vi "Demo - Hardware in the Loop Application.vi"() -> ()   [LabVIEW 2017]
doc: "This application demonstrates the basic application of the hardware in the loop mode.\n\n-Initialises and configures the device\n-Uploads data the arbitrary waveform generator\n-Runs a shot\n-Downloads the data and displays it\n-Changes the data\n-Repeats the process"
uses:
  Communications/Typedefs/Data Size--Enum.ctl
  Communications/Communications Library.lvlib
  GUI/Consoles/Communications Console Library.lvlib
panel:
  in  "Analog In Data Size":T1
  in  "Display Console":bool
  in  "INI File Path":path caption="INI File Path (Blank for Defaults)"
  out "Ready":bool
  out "error out":errorcluster
  out "Number of Shots Run":i32
  in  "stop":bool
  in  "Dynamic Channel":i32
  in  "Speed":dbl=0.5 format="%#_13g"
  out "Data Received":bool
  out "Shot Completed":bool
  in  "Samples to Read":i32=80000
  in  "Length of AO Data (Samples)":i32=32768
  out "Analog Input Plot":i32[][](graph)
  out "Analog Output Plot":i16[][](graph)
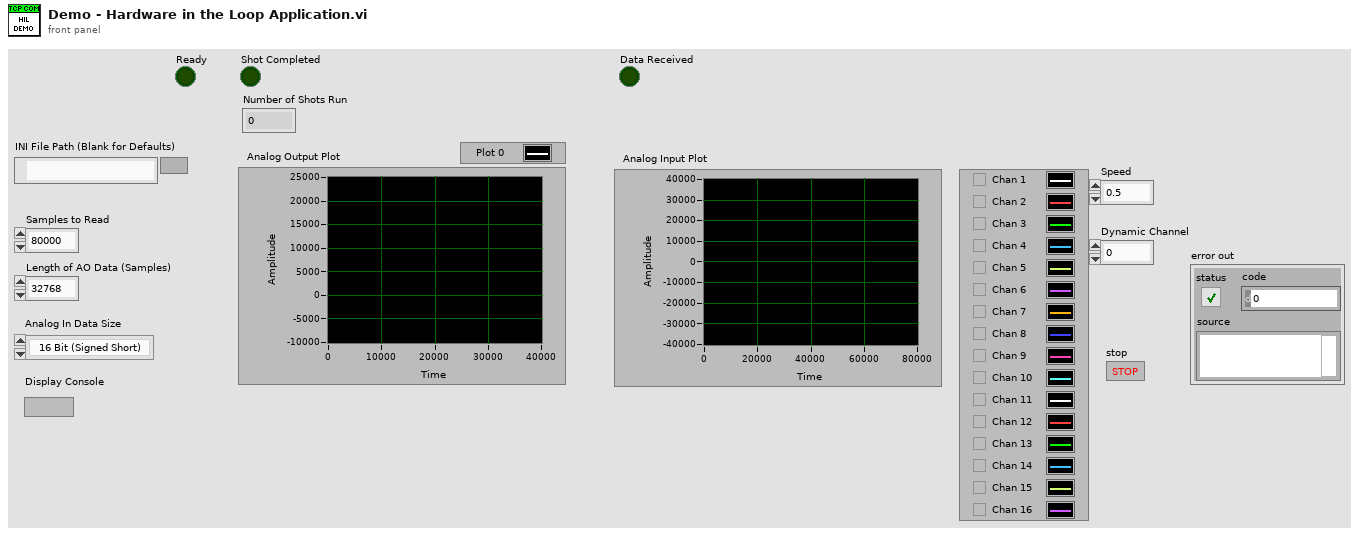
[diagram p1: front panel]
types:
  T1 = typedef "Communications Library.lvlib/Data Size--Enum.ctl" = enum16{"16 Bit (Signed Short)", "32 Bit (Signed Long)"}
  T2 = typedef "Communications Library.lvlib/DTACQ Module Carrier Configuration--Cluster.ctl" = cluster{"Name":string, "IP":string, "Control Port":i32, "Timeout (ms)":i32, "Continuous Capture Port (Multiplexed)":i32, "Start HIL Shot Port":i32, "AWG Upload Port (Multiplexed)":i32, "Download Captured Data Port (Multiplexed)":i32, "Module Slots":i32, "Module Configurations":T3[]}
  T3 = typedef "Communications Library.lvlib/DTACQ Module Configuration--Cluster.ctl" = cluster{"Name":string, "Position":string, "Module Type":T4, "Control Port":i32, "Timeout (ms)":i32, "Channels":i32}
  T4 = typedef "Communications Library.lvlib/DTACQ Device Type--Enum.ctl" = enum16{"Carrier", "Analog In Module", "Analog Out Module", "Generic Module"}
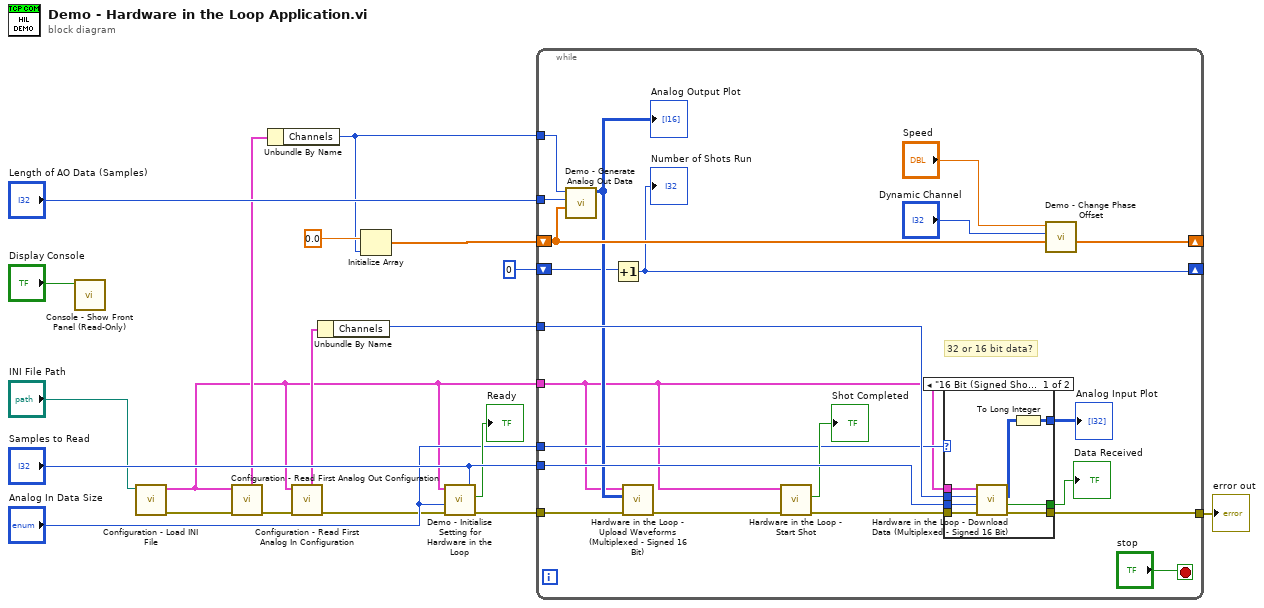
[diagram p0: block diagram]
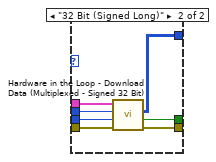
[diagram p2: hidden frame]
diagram:
  n1 = call "Console - Show Front Panel (Read-Only).vi"("Display Console"="Display Console") -> ()  [unwired: 11 in]
  n2 = call "Configuration - Load INI File.vi"("configuration file path"="INI File Path") -> ("error out"=w12:errorcluster, "Carrier Configuration Out"=w1:T2)  [unwired: 9 in]
  n3 = call "Configuration - Read First Analog Out Configuration.vi"("error in"=w12, "Configuration Cluster"=w1) -> ("error out"=w11:errorcluster, "AO - Module Configuration"=w10:T3)  [unwired: 5 in, 3 out]
  n4 = Unbundle By Name(w10) -> ("Channels"=w9:i32)
  n5 = call "Configuration - Read First Analog In Configuration.vi"("error in"=w11, "Carrier Configuration"=w1) -> ("error out"=w2:errorcluster, "AI - Module Configuration"=w8:T3)  [unwired: 5 in, 3 out]
  n6 = Unbundle By Name(w8) -> ("Channels"=w7:i32)
  n7 = Initialize Array(0.0, w9) -> (w17:dbl[])
  n8 = call "Demo - Initialise Setting for Hardware in the Loop.vi"("error in"=w2, "Analog In Data Size"="Analog In Data Size", "Samples to Read"="Samples to Read", "Carrier Configuration"=w1) -> ("error out"=w5:errorcluster, "Ready"=→"Ready":bool)  [unwired: 6 in]
  n9 = while {
    tunnel: w1 -> [w20]
    tunnel: w7 -> [w40]
    tunnel: "Samples to Read" -> [w39]
    tunnel: "Length of AO Data (Samples)" -> [w37]
    tunnel: w9 -> [w38]
    shift-right: [w33] -> _
    shift-left: w17 -> [w34]
    tunnel: [w35] -> w18
    shift-right: [w30] -> _
    shift-left: 0 -> [w31]
    tunnel: w5 -> [w29]
    tunnel: "Analog In Data Size" -> [w22]
    stop <- "stop" stop-if-true
    # "32 or 16 bit data?"
    n10 = call "Demo - Generate Analog Out Data.vi"("Phase Offset (Radians)"=w34, "Number of Samples"=w37, "Number of AO Channels"=w38) -> ("Sine Wave"=w32:i16[][])  [unwired: 8 in]
    "Analog Output Plot" <- w32
    n11 = Increment(x=w31) -> (x+1=w30:i32)
    "Number of Shots Run" <- w30
    n12 = call "Hardware in the Loop - Upload Waveforms (Multiplexed - Signed 16 Bit).vi"("error in"=w29, "Multichannel Waveform"=w32, "Configuration Cluster"=w20) -> ("error out"=w26:errorcluster)  [unwired: 8 in]
    n13 = call "Hardware in the Loop - Start Shot.vi"("error in"=w26, "Configuration Cluster"=w20) -> ("error out"=w25:errorcluster, "Shot Completed"=→"Shot Completed":bool)  [unwired: 8 in]
    n14 = case shown="\"16 Bit (Signed Short)\", Default" w22 {
      tunnel: w40 -> [w48 w50]
      tunnel: w39 -> [w47 w49]
      tunnel: [w46 w54] -> w35
      tunnel: w20 -> [w45 w51]
      tunnel: w25 -> [w44 w55]
      tunnel: [w43 w53] -> w23
      tunnel: [w41 w52] -> w21
      frame "16 Bit (Signed Short)", Default {
        n15 = call "Hardware in the Loop - Download Data (Multiplexed - Signed 16 Bit).vi"("error in"=w44, "Number of Samples"=w47, "Number of Channels"=w48, "Configuration Cluster"=w45) -> ("error out"=w46:errorcluster, "Data Received"=w43:bool, "Data"=w42:i16[][])  [unwired: 5 in]
        n16 = To Long Integer(number=w42) -> (32bit integer=w41:i32[][])
      }
      frame "32 Bit (Signed Long)" {
        n17 = call "Hardware in the Loop - Download Data (Multiplexed - Signed 32 Bit).vi"("error in"=w55, "Number of Samples"=w49, "Number of Channels"=w50, "DTACQ Module Carrier Configuration"=w51) -> ("error out"=w54:errorcluster, "Data Received"=w53:bool, "Data"=w52:i32[][])  [unwired: 5 in]
      }
    }
    "Analog Input Plot" <- w21
    "Data Received" <- w23
    n18 = call "Demo - Change Phase Offset.vi"("Phase Offset (Radians) in"=w34, "Channel"="Dynamic Channel", "x"="Speed") -> ("Phase Offset (Radians) out"=w33:dbl[])  [unwired: 8 in]
  }
  "error out" <- w18
